vi "SignalMeasurements_TU.vi"() -> ()   [LabVIEW 2025]
uses:
  <vilib>/measure/NI_MABase.lvlib
panel:
  out "error out":errorcluster
  out "max frequency":dbl
  out "signal power":dbl
  out "f0":dbl
  out "df":dbl
  out "magnitude":dbl[](graph)
  in  "error in":errorcluster
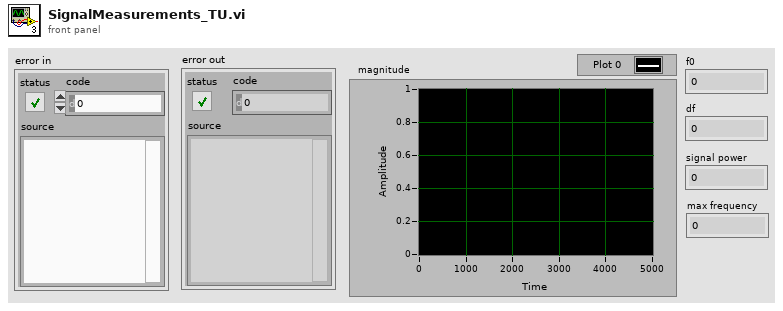
[diagram p1: front panel]
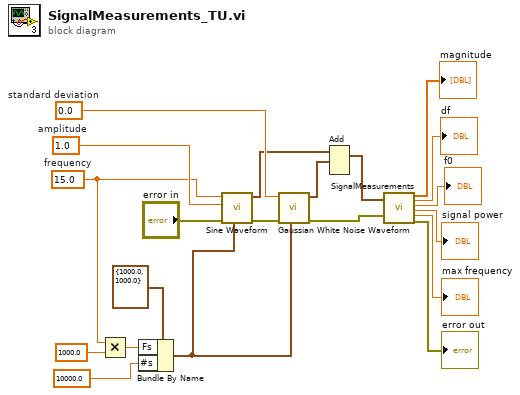
[diagram p0: block diagram]
diagram:
  w8 = 15.0  # frequency
  w14 = 1.0  # amplitude
  w12 = 0.0  # standard deviation
  n1 = Multiply(x=w8, y=1000.0) -> (x*y=w7:dbl)
  n2 = Bundle By Name(cluster=cluster{"Fs":dbl, "#s":dbl} {"Fs"=1000.0, "#s"=1000.0} ("sampling info"), "Fs"=w7, "#s"=10000.0) -> (w5:cluster{"Fs":dbl, "#s":dbl})
  n3 = call <vilib>:"Sine Waveform.vi"("sampling info"=w5, "error in (no error)"="error in", "amplitude"=w14, "frequency"=w8) -> ("error out"=w13:errorcluster, "signal out"=w2:waveform(dbl))  [unwired: 6 in]
  n4 = call <vilib>:"Gaussian White Noise Waveform.vi"("sampling info"=w5, "error in (no error)"=w13, "standard deviation"=w12) -> ("error out"=w4:errorcluster, "signal out"=w3:waveform(dbl))  [unwired: 7 in]
  n5 = Add(1:w3, 2:w2) -> (0:w1:waveform(dbl))  [unwired: 1 in, 1 out]
  n6 = call "SignalMeasurements.vi"("Waveform"=w1, "error in"=w4) -> ("magnitude"=→"magnitude":dbl[], "df"=→"df":dbl, "f0"=→"f0":dbl, "signal power"=→"signal power":dbl, "max frequency"=→"max frequency":dbl, "error out"=→"error out":errorcluster)  [unwired: 12 in]
